vi "Read Paths.vi"(8 "error in (no error)":errorcluster, 11 "Cable Path Group in":refnum<class "Path Group.lvclass">) -> (0 "error out":errorcluster, 2 "Paths":refnum<class "Path.lvclass">[](array[class]), 3 "Cable Path Group out":refnum<class "Path Group.lvclass">)   [LabVIEW 2023, in "RFCalAndFixtureCharact.Common.lvlib" / "Path Group.lvclass"]
uses:
  Path Group.lvclass
  Path/Path.lvclass
  Path Group.lvclass/Path Group.ctl
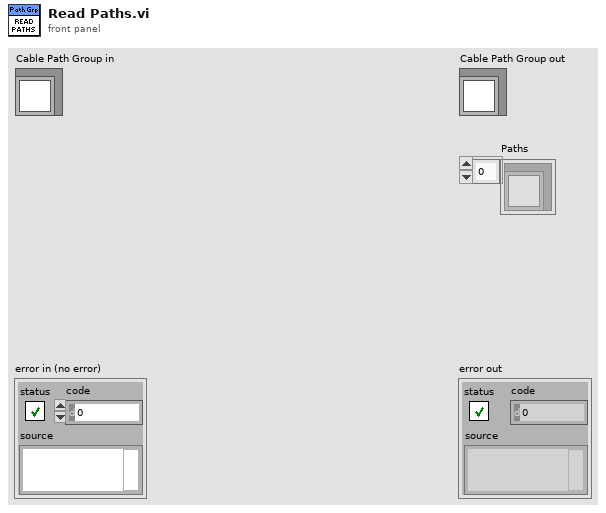
[diagram p1: front panel]
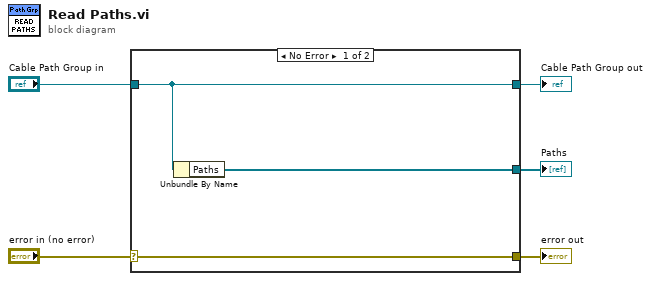
[diagram p0: block diagram]
diagram:
  n1 = case shown="No Error" "error in (no error)" {
    selector: "error in (no error)" -> [w8 w9]
    tunnel: [w8 w9] -> w4
    tunnel: [w7 w10] -> w2
    tunnel: "Cable Path Group in" -> [w7 w10]
    tunnel: [w6 _] -> w1
    frame No Error {
      n2 = Unbundle By Name(w7) -> ("Paths"=w6:refnum<class "Path.lvclass">[])
    }
    frame Error {
    }
  }
  "error out" <- w4
  "Cable Path Group out" <- w2
  "Paths" <- w1
